vi "Teleop.vi"(10 "Match Info":T1={"Autonomous Elapsed Seconds"=0.0, "TeleOp Elapsed Seconds"=0.0, "Disabled Elapsed Seconds"=0.0, "Visited Autonomous"=FALSE, "Visited TeleOp"=FALSE, "Visited Disabled"=FALSE, "Autonomous Settings"={"Autonomous Style"=enum."Independent", "VI Refnum"=refnum}}, 11 "Call Context":T2) -> ()   [LabVIEW 2016]
doc: "This VI is called for each TeleOp packet received from the DS where the robot is not disabled. It is often used to read from the joysticks and update I/O or to update setpoints for timed control loops. It should complete and return within 20 milliseconds or it may miss DS packets."
uses:
  <vilib>/Rock Robotics/WPI/DriverStation/WPI_DriverStationDerivedRobotMode.ctl
  <vilib>/Rock Robotics/WPI/DriverStation/WPI_DriverStationMatch Info.ctl
  <vilib>/Rock Robotics/WPI/Utilities/WPI_GetSetVariantRefNum.vi
  <vilib>/Rock Robotics/Network Tables/NT Write Boolean Array.vi
  <vilib>/Rock Robotics/Network Tables/NT Write Numeric Array.vi
  <vilib>/Rock Robotics/Network Tables/NT Read Boolean.vi
  <vilib>/Rock Robotics/Network Tables/NT Read Number.vi
  Robot Global Data.vi
panel:
  in  "Drive Mode":enum16{"Tank Drive", "Arcade Drive"}(ring)
  in  "Controller Mode":enum16{"X-Box Controller", "Joysticks"}(ring)
  out "Sample Slider 0":dbl(slide) scale=0.0..5.0
  out "Sample Boolean 1":bool
  out "Sample Boolean 0":bool
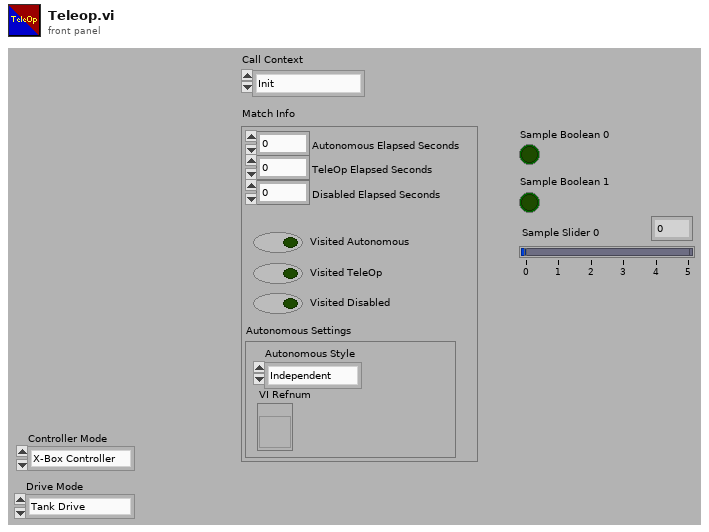
[diagram p1: front panel]
types:
  T1 = typedef "WPI_DriverStationMatch Info.ctl" = cluster{"Autonomous Elapsed Seconds":dbl, "TeleOp Elapsed Seconds":dbl, "Disabled Elapsed Seconds":dbl, "Visited Autonomous":bool, "Visited TeleOp":bool, "Visited Disabled":bool, "Autonomous Settings":cluster{"Autonomous Style":enum16{"Iterative", "Independent"}, "VI Refnum":refnum<vi>}}
  T2 = typedef "WPI_DriverStationDerivedRobotMode.ctl" = enum16{"Init", "Execute", "Stop"}
  T3 = typedef "WPI_JoystickDevRef.ctl" = cluster{"Device":T4}
  T4 = typedef "WPI_JoystickDeviceEnum.ctl" = enum16{"USB 0", "USB 1", "USB 2", "USB 3", "USB 4", "USB 5"}
  T5 = typedef "WPI_RobotDriveDevRef.ctl" = cluster{"DevStatus":errorcluster, "Motors[]":T6[], "Square Inputs":bool, "Max Output":dbl}
  T6 = typedef "WPI_MotorControlDeviceRef.ctl" = cluster{"DeviceStatus":errorcluster, "Type":T7, "PWM":cluster{"PWM Channel":T8, "DeadBand":T9}, "CAN":cluster{"Device Number":u8, "SetOutput VI Ref":variant, "GetOutput VI Ref":variant, "Enable VI Ref":variant, "Disable VI Ref":variant, "Data":variant}, "Invert":bool}
  T7 = typedef "WPI_MotorControlType.ctl" = enum16{"PWM", "CAN"}
  T8 = typedef "FPGA_DIOPWMChannel.ctl" = enum8{"PWM 0", "PWM 1", "PWM 2", "PWM 3", "PWM 4", "PWM 5", "PWM 6", "PWM 7", "PWM 8", "PWM 9", "PWM MXP 0", "PWM MXP 1", "PWM MXP 2", "PWM MXP 3", "PWM MXP 4", "PWM MXP 5", "PWM MXP 6", "PWM MXP 7", "PWM MXP 8", "PWM MXP 9", "Invalid"}
  T9 = typedef "WPI_PWMDeadband.ctl" = cluster{"Name":string, "maxPositivePwm":i32, "minPositivePwm":i32, "centerPwm":i32, "maxNegativePwm":i32, "minNegativePwm":i32, "angularRange":u16}
  T10 = cluster{"Current Position":enum16{"Down", "Up"}, "Current State":enum16{"Down", "Shifting", "Up"}}
  T11 = cluster{"Current Position":enum16{"Closed", "Open"}, "Current State":enum16{"Closed", "Shifting", "Open"}}
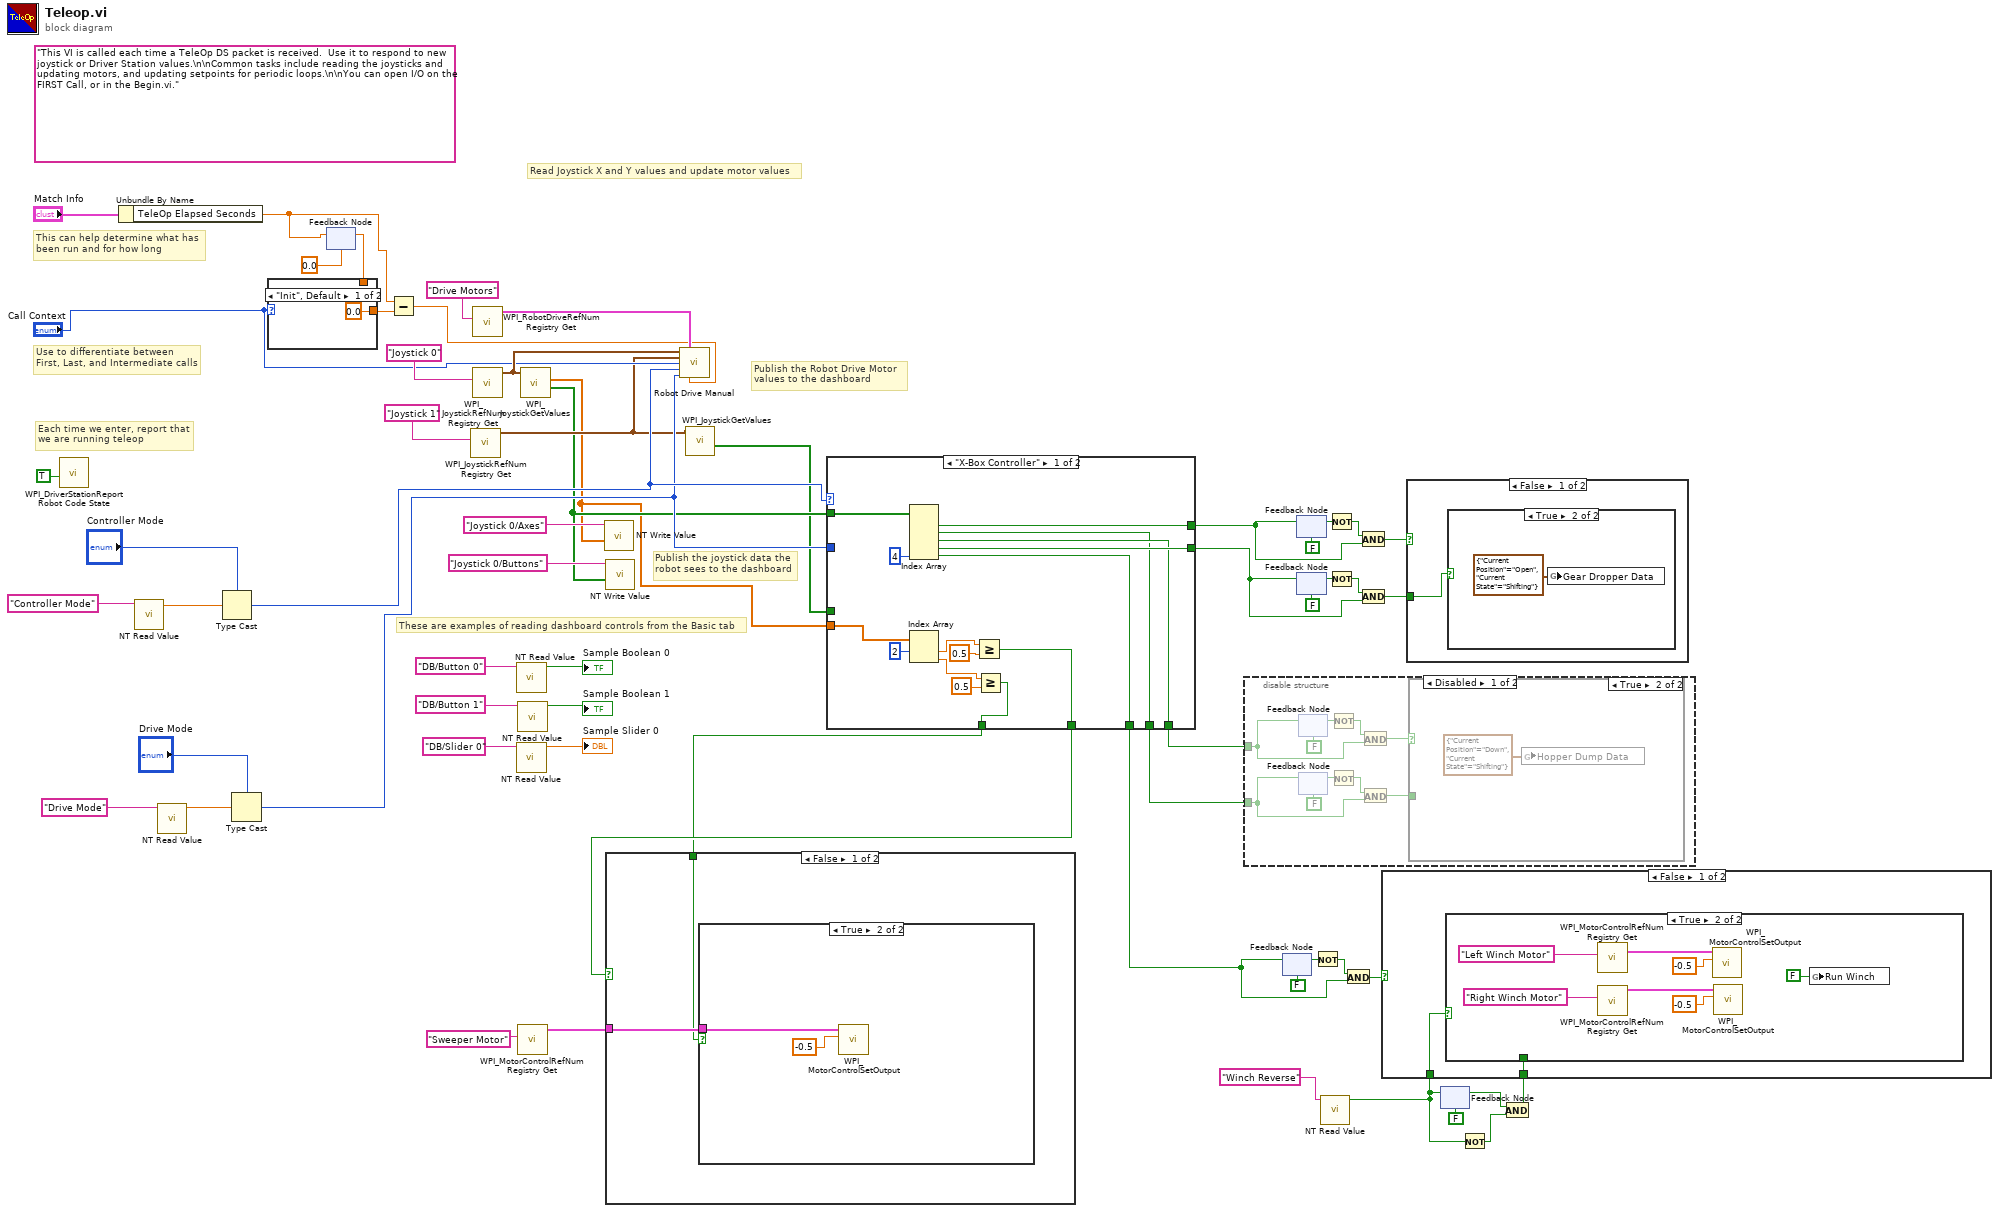
[diagram p0: block diagram]
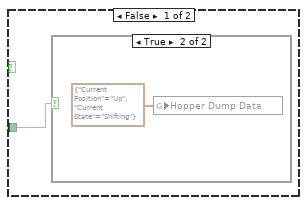
[diagram p2: hidden frame]
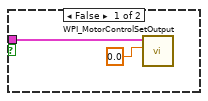
[diagram p5: hidden frame]
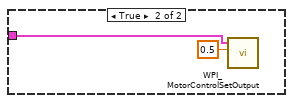
[diagram p6: hidden frame]
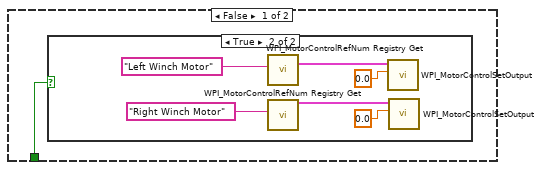
[diagram p7: hidden frame]
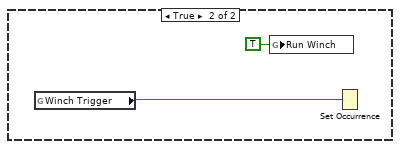
[diagram p9: hidden frame]
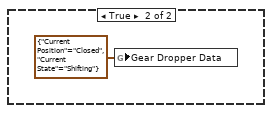
[diagram p11: hidden frame]
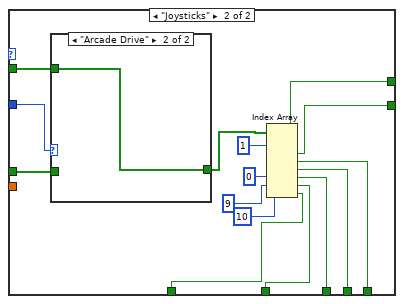
[diagram p12: hidden frame]
diagram:
  (unwired) "This VI is called each time a TeleOp DS packet is received.  Use it to respond to new joystick or Driver Station values.\n\nCommon tasks include reading the joysticks and updating motors, and updating setpoints for periodic loops.\n\nYou can open I/O on the FIRST Call, or in the Begin.vi."
  # "These are examples of reading dashboard controls from the Basic tab"
  # "Publish the Robot Drive Motor\nvalues to the dashboard"
  # "Publish the joystick data the\nrobot sees to the dashboard"
  # "Each time we enter, report that\nwe are running teleop"
  # "Use to differentiate between\nFirst, Last, and Intermediate calls"
  # "This can help determine what has\nbeen run and for how long"
  # "Read Joystick X and Y values and update motor values"
  n1 = call <vilib>:"WPI_DriverStationReport Robot Code State.vi"("TeleOp"=TRUE ("Autonomous")) -> ()  [unwired: 10 in, 1 out]
  n2 = Unbundle By Name("Match Info") -> ("TeleOp Elapsed Seconds"=w36:dbl)
  n3 = call-poly <vilib>:"NT Read Value.vi"("Name"="Controller Mode") -> ("Numeric"=w43:dbl)  [unwired: 9 in, 1 out]
  n4 = call-poly <vilib>:"NT Read Value.vi"("Name"="Drive Mode") -> ("Numeric"=w41:dbl)  [unwired: 9 in, 1 out]
  n5 = Type Cast(type="Controller Mode", x=w43) -> (*(type *) &x=w33:enum16{"X-Box Controller", "Joysticks"})
  n6 = Type Cast(type="Drive Mode", x=w41) -> (*(type *) &x=w32:enum16{"Tank Drive", "Arcade Drive"})
  n7 = feedback #1(0.0 ("TeleOp Elapsed Seconds")) -> (w38:dbl)
  n8 = case shown="\"Init\", Default" "Call Context" {
    tunnel: w38 -> [_ w62]
    tunnel: [0.0 ("TeleOp Elapsed Seconds") w62] -> w37
    frame "Init", Default {
    }
    frame "Execute" {
    }
  }
  n9 = feedback-in #1(w36) -> ()
  n10 = Subtract(x=w36, y=w37) -> (x-y=w35:dbl)
  n11 = call <vilib>:"WPI_JoystickRefNum Registry Get.vi"("refnum name"="Joystick 1") -> ("JoystickDevRef"=w31:T3)  [unwired: 1 in, 9 out]
  n12 = call <vilib>:"WPI_RobotDriveRefNum Registry Get.vi"("refnum name"="Drive Motors") -> ("RobotDriveDevRef"=w48:T5)  [unwired: 1 in, 9 out]
  n13 = call <vilib>:"WPI_JoystickRefNum Registry Get.vi"("refnum name"="Joystick 0") -> ("JoystickDevRef"=w47:T3)  [unwired: 1 in, 9 out]
  n14 = call-poly <vilib>:"NT Read Value.vi"("Name"="DB/Button 0" ("refnum name")) -> ("Boolean"=→"Sample Boolean 0":bool)  [unwired: 9 in, 1 out]
  n15 = call-poly <vilib>:"NT Read Value.vi"("Name"="DB/Slider 0" ("refnum name")) -> ("Numeric"=→"Sample Slider 0":dbl)  [unwired: 9 in, 1 out]
  n16 = call-poly <vilib>:"NT Read Value.vi"("Name"="DB/Button 1" ("refnum name")) -> ("Boolean"=→"Sample Boolean 1":bool)  [unwired: 9 in, 1 out]
  n17 = call <vilib>:"WPI_MotorControlRefNum Registry Get.vi"("refnum name"="Sweeper Motor") -> ("MotorControlDevRef"=w9:T6)  [unwired: 9 in, 1 out]
  n18 = call <vilib>:"WPI_JoystickGetValues.vi"("JoystickDevRef"=w47) -> ("Buttons"=w30:bool[], "Axes"=w7:dbl[])  [unwired: 6 in, 3 out]
  n19 = call-poly <vilib>:"NT Write Value.vi"("Numeric Array"=w7, "Name"="Joystick 0/Axes") -> ()  [unwired: 9 in, 1 out]
  n20 = call-poly <vilib>:"NT Write Value.vi"("Boolean Array"=w30, "Name"="Joystick 0/Buttons") -> ()  [unwired: 9 in, 1 out]
  n21 = call "Robot Drive Manual.vi"("Joystick0DevRef"=w47, "RobotDriveDevRef"=w48, "Joystick1DevRef"=w31, "Call Context"="Call Context", "Controller Mode"=w33, "Drive Mode"=w32, "dt"=w35) -> ()  [unwired: 8 in, 1 out]
  n22 = call <vilib>:"WPI_JoystickGetValues.vi"("JoystickDevRef"=w31) -> ("Buttons"=w19:bool[])  [unwired: 6 in, 4 out]
  n23 = case shown="\"X-Box Controller\"" w33 {
    tunnel: w32 -> [_ w92]
    tunnel: w30 -> [w77 w90]
    tunnel: [w76 w87] -> w26
    tunnel: [w75 w86] -> w22
    tunnel: w19 -> [_ w91]
    tunnel: [w74 w85] -> w18
    tunnel: [w73 w84] -> w17
    tunnel: [w72 w83] -> w13
    tunnel: [w64 w81] -> w10
    tunnel: [w63 w79] -> w8
    tunnel: w7 -> [w70 _]
    frame "X-Box Controller" {
      n24 = Index Array(array=w77, index #5=4 ("index")) -> (element #1=w76:bool, element #2=w73:bool, element #3=w74:bool, element #4=w75:bool, element #5=w72:bool)  [unwired: 4 in]
      n25 = Index Array(array=w70, index #1=2 ("index")) -> (element #1=w68:dbl, element #2=w66:dbl)  [unwired: 1 in]
      n26 = Greater Or Equal?(x=w68, y=0.5) -> (x >= y?=w64:bool)
      n27 = Greater Or Equal?(x=w66, y=0.5) -> (x >= y?=w63:bool)
    }
    frame "Joysticks" {
      n28 = case shown="\"Arcade Drive\"" w92 {
        tunnel: [w93 w94] -> w89
        tunnel: w91 -> [w93 _]
        tunnel: w90 -> [_ w94]
        frame "Tank Drive" {
        }
        frame "Arcade Drive" {
        }
      }
      n29 = Index Array(array=w89, index #1=1 ("index"), index #5=0 ("index"), index #6=9 ("index"), index #7=10 ("index")) -> (element #1=w87:bool, element #2=w86:bool, element #3=w85:bool, element #4=w84:bool, element #5=w83:bool, element #6=w81:bool, element #7=w79:bool)  [unwired: 3 in]
    }
  }
  n30 = case shown="False" w10 {
    tunnel: w9 -> [w96 w101]
    tunnel: w8 -> [w95 _]
    frame False {
      n31 = case shown="True" w95 {
        tunnel: w96 -> [w97 w99]
        frame False {
          n32 = call <vilib>:"WPI_MotorControlSetOutput.vi"("Output"=0.0, "MotorControlDevRef"=w97) -> ()  [unwired: 7 in, 3 out]
        }
        frame True {
          n33 = call <vilib>:"WPI_MotorControlSetOutput.vi"("Output"=-0.5, "MotorControlDevRef"=w99) -> ()  [unwired: 7 in, 3 out]
        }
      }
    }
    frame True {
      n34 = call <vilib>:"WPI_MotorControlSetOutput.vi"("Output"=0.5, "MotorControlDevRef"=w101) -> ()  [unwired: 7 in, 3 out]
    }
  }
  n35 = disable-structure shown="Disabled" {
    disable-tunnel: w18 -> [w104 _]
    disable-tunnel: w17 -> [w103 _]
    frame Disabled {
      n36 = feedback #2(FALSE) -> (w111:bool)
      n37 = feedback-in #2(w104) -> ()
      n38 = feedback #3(FALSE) -> (w108:bool)
      n39 = feedback-in #3(w103) -> ()
      n40 = Not(x=w111) -> (.not. x?=w112:bool)
      n41 = Not(x=w108) -> (.not. x?=w109:bool)
      n42 = And(x=w112, y=w104) -> (x .and. y?=w106:bool)
      n43 = And(x=w109, y=w103) -> (x .and. y?=w105:bool)
      n44 = case shown="True" w106 {
        tunnel: w105 -> [w113 _]
        frame False {
          n45 = case shown="True" w113 {
            frame False {
            }
            frame True {
              n46 = global write "Robot Global Data.vi" "Hopper Dump Data"(T10 {"Current Position"=enum."Up", "Current State"=enum."Shifting"} ("Gear Dropper Data")) -> ()
            }
          }
        }
        frame True {
          n47 = global write "Robot Global Data.vi" "Hopper Dump Data"(T10 {"Current Position"=enum."Down", "Current State"=enum."Shifting"} ("Gear Dropper Data")) -> ()
        }
      }
    }
    frame Enabled {
    }
  }
  n48 = feedback #4(FALSE) -> (w15:bool)
  n49 = feedback-in #4(w13) -> ()
  n50 = feedback #5(FALSE) -> (w28:bool)
  n51 = feedback-in #5(w26) -> ()
  n52 = feedback #6(FALSE) -> (w24:bool)
  n53 = feedback-in #6(w22) -> ()
  n54 = Not(x=w15) -> (.not. x?=w16:bool)
  n55 = call-poly <vilib>:"NT Read Value.vi"("Name"="Winch Reverse") -> ("Boolean"=w2:bool)  [unwired: 9 in, 1 out]
  n56 = Not(x=w28) -> (.not. x?=w29:bool)
  n57 = Not(x=w24) -> (.not. x?=w25:bool)
  n58 = And(x=w16, y=w13) -> (x .and. y?=w12:bool)
  n59 = And(x=w29, y=w26) -> (x .and. y?=w21:bool)
  n60 = And(x=w25, y=w22) -> (x .and. y?=w20:bool)
  n61 = case shown="False" w21 {
    tunnel: w20 -> [w116 _]
    frame False {
      n62 = case shown="True" w116 {
        frame False {
        }
        frame True {
          n63 = global write "Robot Global Data.vi" "Gear Dropper Data"(T11 {"Current Position"=enum."Open", "Current State"=enum."Shifting"} ("Gear Dropper Data")) -> ()
        }
      }
    }
    frame True {
      n64 = global write "Robot Global Data.vi" "Gear Dropper Data"(T11 {"Current Position"=enum."Closed", "Current State"=enum."Shifting"} ("Gear Dropper Data")) -> ()
    }
  }
  n65 = feedback #7(FALSE) -> (w3:bool)
  n66 = feedback-in #7(w2) -> ()
  n67 = Not(x=w2) -> (.not. x?=w5:bool)
  n68 = And(x=w3, y=w5) -> (x .and. y?=w1:bool)
  n69 = case shown="False" w12 {
    tunnel: w2 -> [w120 _]
    tunnel: w1 -> [w119 _]
    frame False {
      n70 = case shown="True" w120 {
        tunnel: w119 -> [w121 _]
        frame False {
          n71 = case shown="True" w121 {
            frame False {
            }
            frame True {
              n72 = call <vilib>:"WPI_MotorControlRefNum Registry Get.vi"("refnum name"="Left Winch Motor") -> ("MotorControlDevRef"=w123:T6)  [unwired: 9 in, 1 out]
              n73 = call <vilib>:"WPI_MotorControlRefNum Registry Get.vi"("refnum name"="Right Winch Motor") -> ("MotorControlDevRef"=w122:T6)  [unwired: 9 in, 1 out]
              n74 = call <vilib>:"WPI_MotorControlSetOutput.vi"("Output"=0.0, "MotorControlDevRef"=w123) -> ()  [unwired: 7 in, 3 out]
              n75 = call <vilib>:"WPI_MotorControlSetOutput.vi"("Output"=0.0, "MotorControlDevRef"=w122) -> ()  [unwired: 7 in, 3 out]
            }
          }
        }
        frame True {
          n76 = call <vilib>:"WPI_MotorControlRefNum Registry Get.vi"("refnum name"="Left Winch Motor") -> ("MotorControlDevRef"=w129:T6)  [unwired: 9 in, 1 out]
          n77 = call <vilib>:"WPI_MotorControlRefNum Registry Get.vi"("refnum name"="Right Winch Motor") -> ("MotorControlDevRef"=w128:T6)  [unwired: 9 in, 1 out]
          n78 = call <vilib>:"WPI_MotorControlSetOutput.vi"("Output"=-0.5, "MotorControlDevRef"=w129) -> ()  [unwired: 7 in, 3 out]
          n79 = call <vilib>:"WPI_MotorControlSetOutput.vi"("Output"=-0.5, "MotorControlDevRef"=w128) -> ()  [unwired: 7 in, 3 out]
          n80 = global write "Robot Global Data.vi" "Run Winch"(FALSE ("Run Winch")) -> ()
        }
      }
    }
    frame True {
      n81 = global read "Robot Global Data.vi" "Winch Trigger"() -> (w136:refnum<k4>)
      n82 = global write "Robot Global Data.vi" "Run Winch"(TRUE ("Run Winch")) -> ()
      n83 = Set Occurrence(w136) -> ()
    }
  }
